vi "DistributedCSMModule.vi"(7 "Name(\"\" to use uuid)":string="Event CSM") -> ()   [LabVIEW 2020]
uses:
  <userlib>/_NEVSTOP/Communicable State Machine(CSM)/_Support/Common/Format Timestamp.vi
  <userlib>/_NEVSTOP/Communicable State Machine(CSM)/AdvanceAPI/CSM - Revert Arguments-Safe String.vi
  <userlib>/_NEVSTOP/Communicable State Machine(CSM)/_Support/Common/Trim Single line Text.vi
  <userlib>/_NEVSTOP/Communicable State Machine(CSM)/AdvanceAPI/CSM - Make String Arguments Safe.vi
  <userlib>/_NEVSTOP/Communicable State Machine(CSM)/AdvanceAPI/CSM - Break Down Multiple States String.vi
  <userlib>/_NEVSTOP/Communicable State Machine(CSM)/AdvanceAPI/CSM - Compact Multiple States.vi
  <userlib>/_NEVSTOP/Communicable State Machine(CSM)/AdvanceAPI/CSM - Keywords.vi
  <userlib>/_NEVSTOP/Communicable State Machine(CSM)/_Support/CSMQ/_CSMOFGV.vi
  <userlib>/_NEVSTOP/Communicable State Machine(CSM)/Communicable State Machine.lvlib
panel:
  out "State History":string
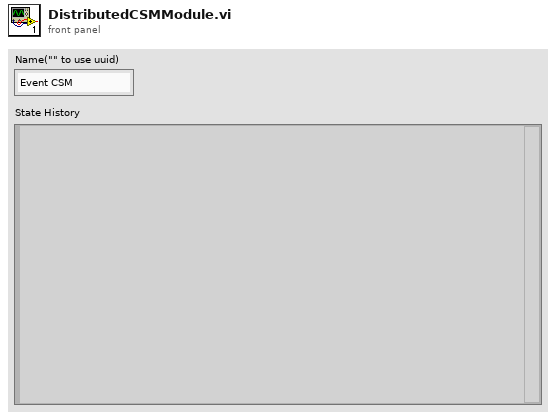
[diagram p1: front panel]
types:
  T1 = enum32{"Invalid", "Standard", "Closed", "Hidden", "Minimized", "Maximized"}
  T2 = enum32{"invalid app kind", "Development System", "Run Time System", "Student Edition", "Embedded LabVIEW", "Evaluation", "Custom"}
  T3 = typedef "Communicable State Machine.lvlib/_CSM_Response Source Message.ctl" = cluster{"‘State":string, "’Arguments":string, "’Error":errorcluster}
  T4 = cluster{"Current VI Reference":refnum<vi>, "Close Panel on Exit?":bool}
  T5 = cluster{"Core":cluster{"Current VI Reference":refnum<vi>, "Close Panel on Exit?":bool}, "Your Boolean data":bool, "Your string data":string}
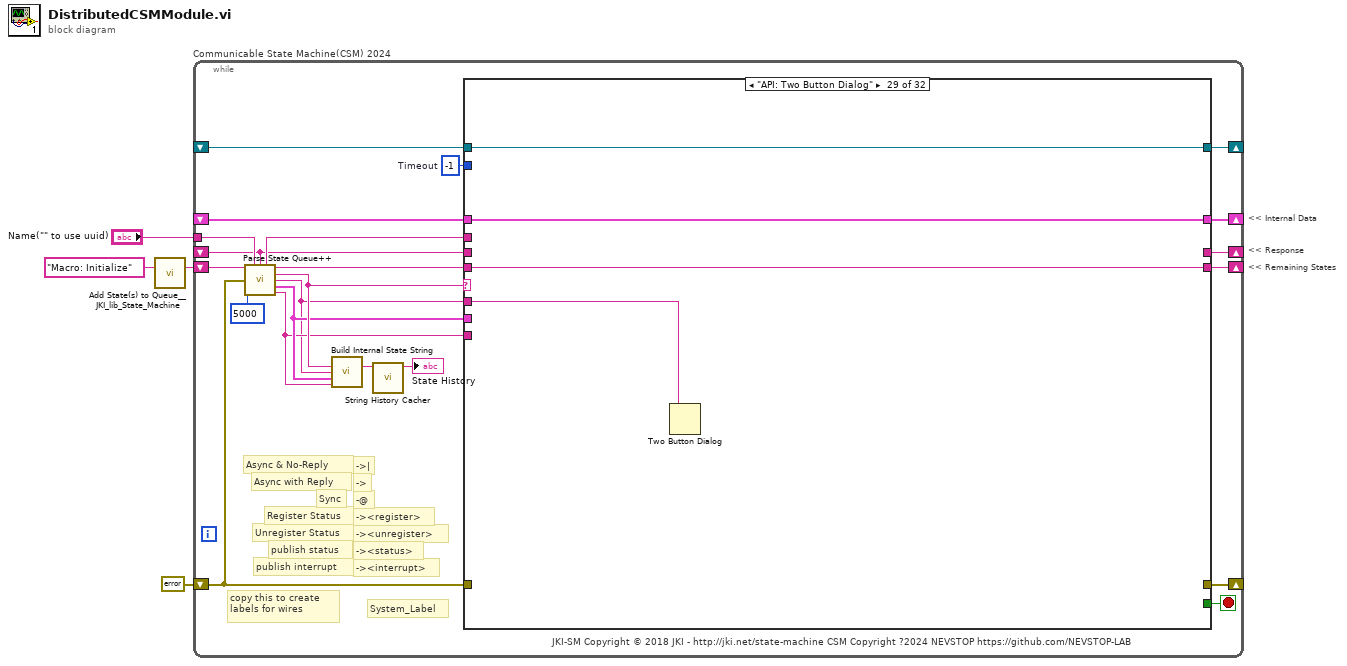
[diagram p0: block diagram]
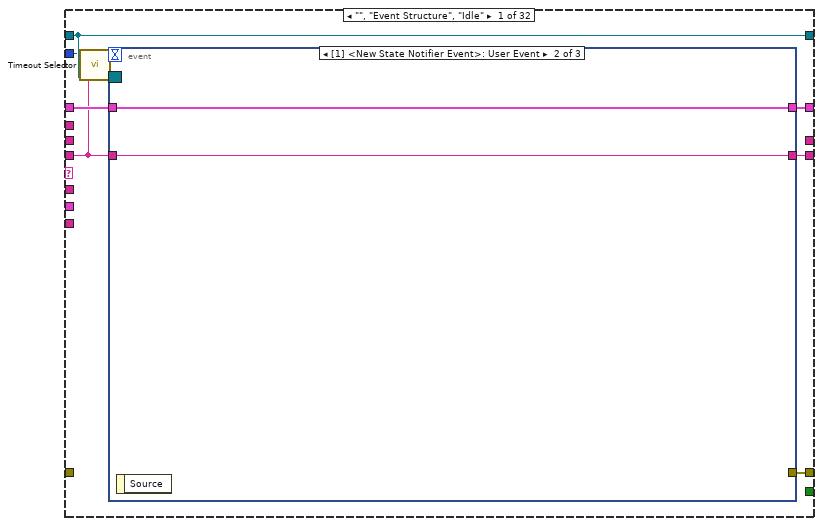
[diagram p2: hidden frame]
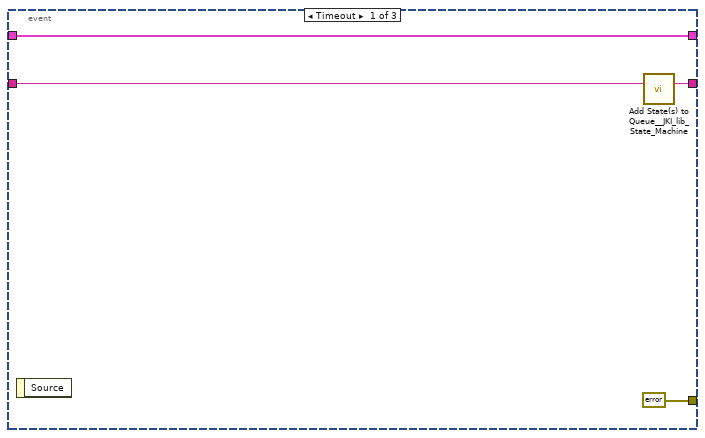
[diagram p3: hidden frame]
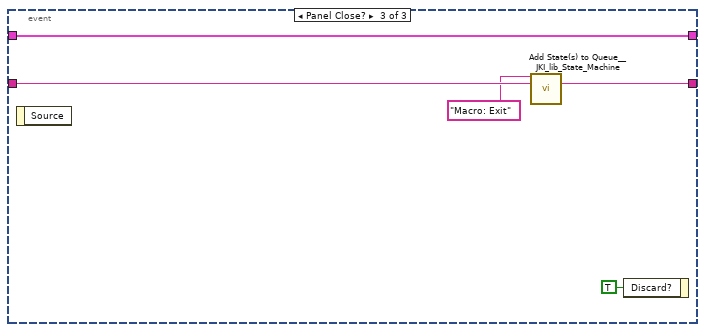
[diagram p4: hidden frame]
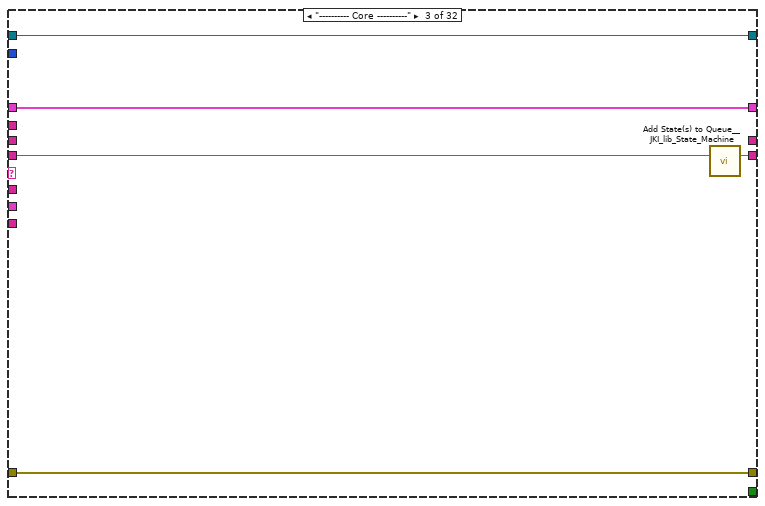
[diagram p6: hidden frame]
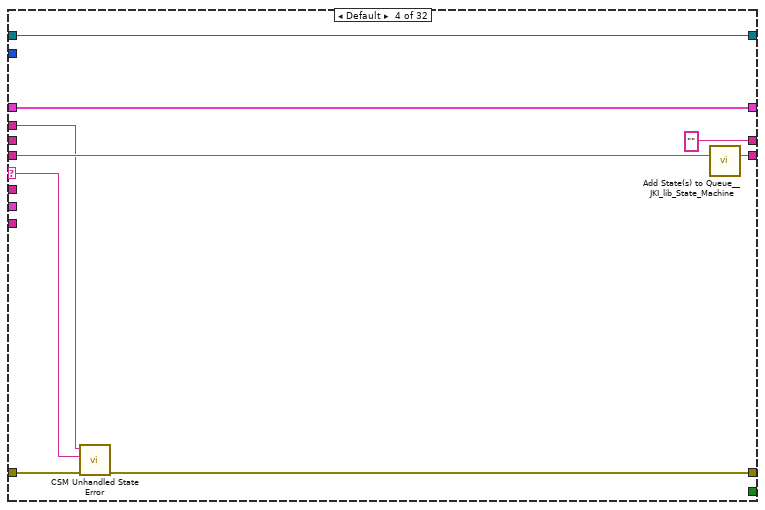
[diagram p7: hidden frame]
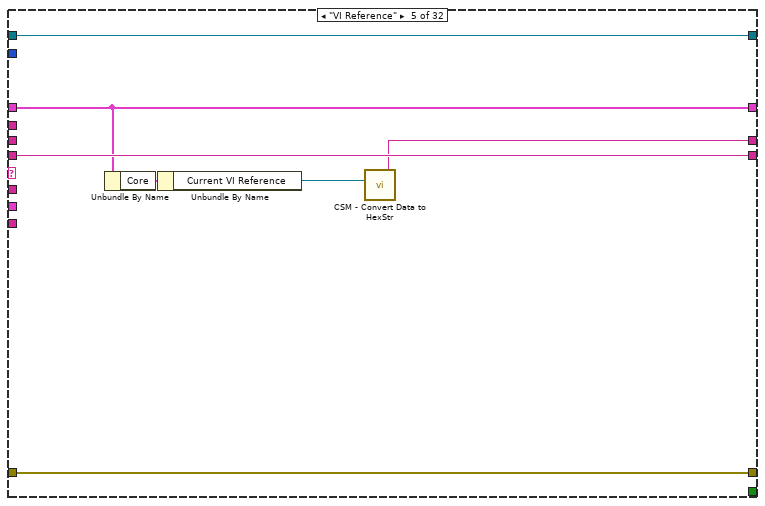
[diagram p8: hidden frame]
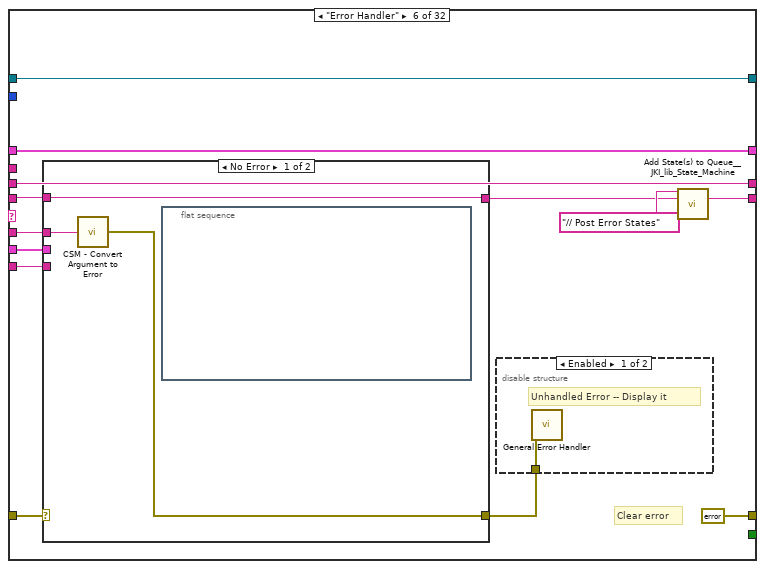
[diagram p9: hidden frame]
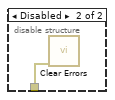
[diagram p10: hidden frame]
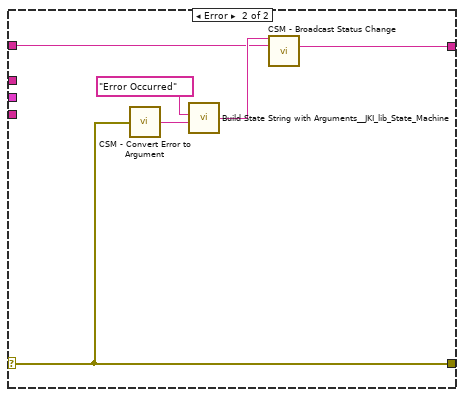
[diagram p11: hidden frame]
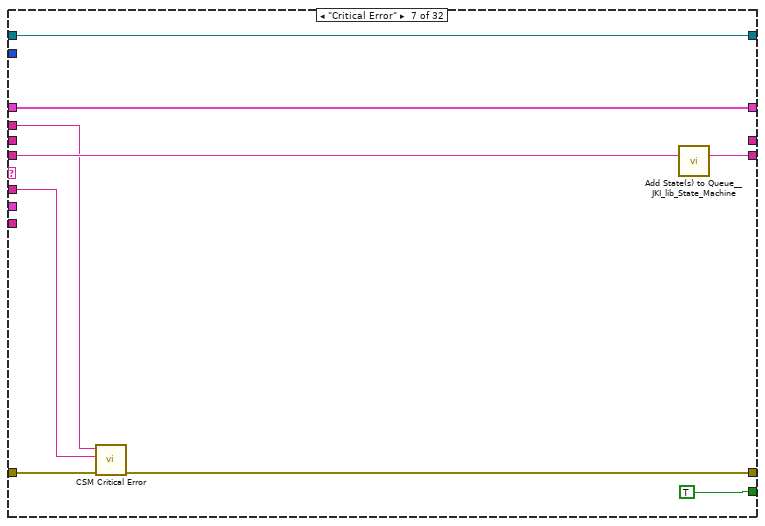
[diagram p12: hidden frame]
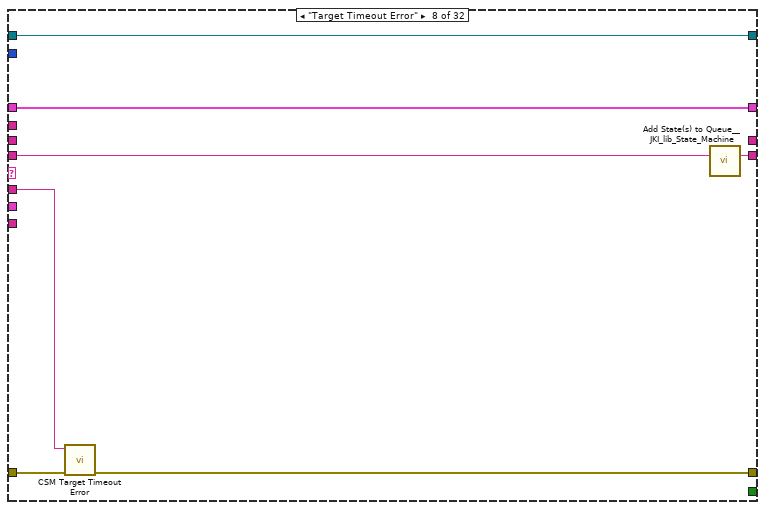
[diagram p13: hidden frame]
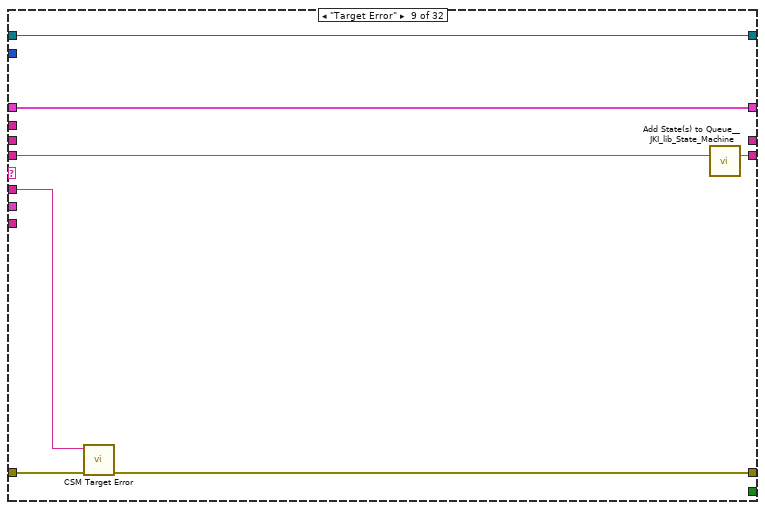
[diagram p14: hidden frame]
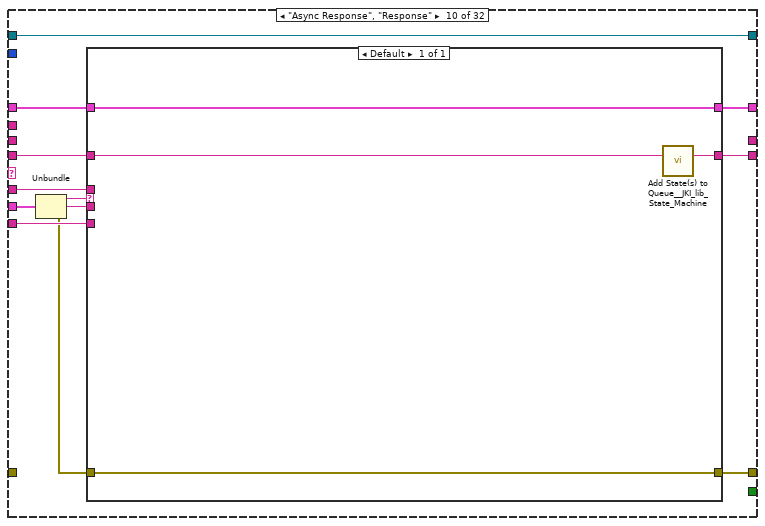
[diagram p15: hidden frame]
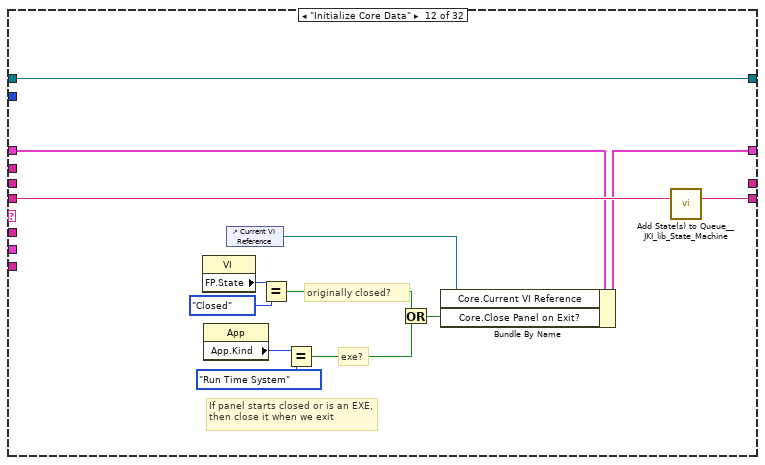
[diagram p17: hidden frame]
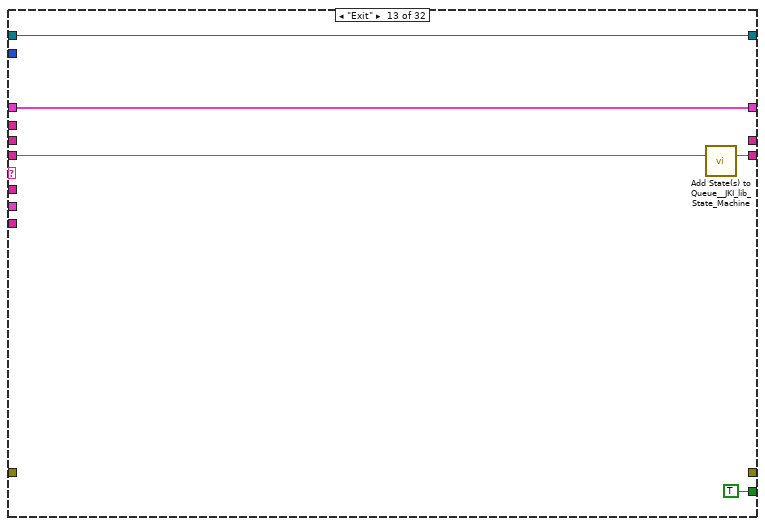
[diagram p18: hidden frame]
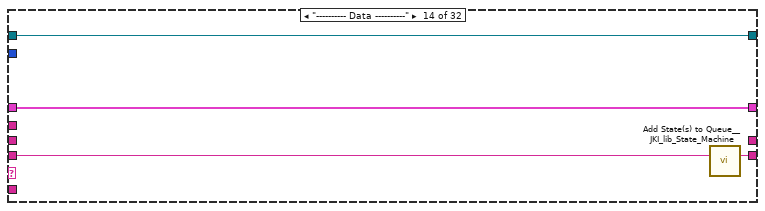
[diagram p19: hidden frame]
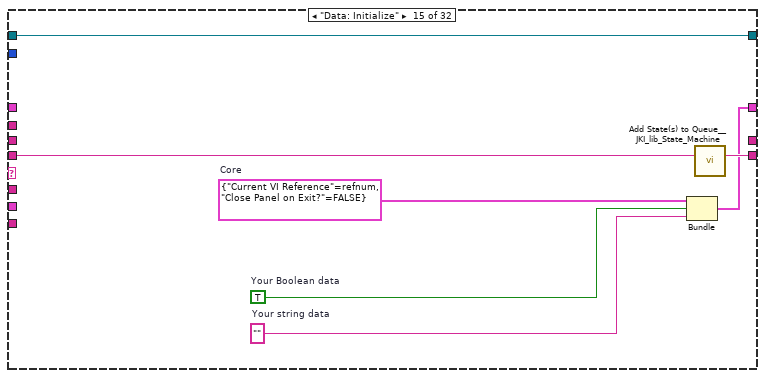
[diagram p20: hidden frame]
diagram:
  # "<< Internal Data"
  # "<< Response"
  # "<< Remaining States"
  n1 = call <vilib>:"Add State(s) to Queue__JKI_lib_State_Machine.vi"("State(s) in (\"\")"="Macro: Initialize" ("Init State(\"Macro: Initialize\")")) -> ("States Out"=w1:string)  [unwired: 14 in]
  n2 = while "Communicable State Machine(CSM) 2024" {
    shift-right: [w21] -> _
    shift-left: _ -> [w20]
    shift-right: [w24] -> _
    shift-left: errorcluster {"status"=FALSE, "code"=0, "source"=""} ("error out") -> [w18]
    shift-right: [w23] -> _
    shift-left: w1 -> [w25]
    tunnel: "Name(\"\" to use uuid)" -> [w13]
    shift-right: [w16] -> _
    shift-left: _ -> [w6]
    shift-right: [w15] -> _
    shift-left: _ -> [w14]
    stop <- w22 stop-if-true
    w19 = -1  # Timeout
    # "-><interrupt>"
    # "-><status>"
    # "-><unregister>"
    # "-><register>"
    # "-@"
    # "->"
    # "->|"
    # "publish interrupt"
    # "publish status"
    # "Unregister Status"
    # "Register Status"
    # "Sync"
    # "Async with Reply"
    # "Async & No-Reply"
    # "copy this to create labels for wires"
    # "System_Label"
    # "JKI-SM Copyright © 2018 JKI - http://jki.net/state-machine CSM Copyright ?2024 NEVSTOP https://github.com/NEVSTOP-LAB"
    n3 = call <userlib>:"Parse State Queue++.vi"("State Queue"=w25, "Name(\"\" to use uuid)"=w13, "Response Arguments"=w6, "Error In (no error)"=w18, "Response Timeout(5000ms)"=5000 ("Response Timeout(1000ms)")) -> ("Name Used"=w7:string, "Remaining States"=w26:string, "Current State"=w10:string, "Arguments"=w5:string, ">> Response Source Message >>"=w9:T3, ">> Source CSM >>"=w8:string)  [unwired: 5 in]
    n4 = call <userlib>:"Build Internal State String.vi"("State"=w10, "Arguments (\"\")"=w5, ">> Response Source Message >>"=w9, "Source (\"\")"=w8) -> ("State with Arguments"=w11:string)  [unwired: 11 in]
    n5 = call <userlib>:"String History Cacher.vi"("String"=w11) -> ("String Cache"=→"State History":string)  [unwired: 10 in]
    n6 = case shown="\"API: Two Button Dialog\"" w10 {
      selector: w10 -> [_ _ _ w56 _ _ _ _ _ _ _ _ _ _ _ _ _ _ _ _ _ _ _ _ _ _ _ _ _ _ _ _]
      tunnel: w26 -> [w27 w48 w53 w62 w68 w75 w101 w109 w116 w126 w135 w148 w153 w157 w164 w170 w174 w181 w185 w189 w193 w199 w211 w275 w280 w291 w294 w298 w302 w306 w310 w314]
      tunnel: w5 -> [_ _ _ _ _ w73 w97 w104 w112 w120 _ _ _ _ _ _ _ _ _ _ _ w195 w206 _ _ _ _ w295 w299 _ _ _]
      tunnel: w20 -> [w33 w47 w50 w60 w67 w81 w102 w107 w114 w124 w134 w142 w151 w155 _ w166 w172 w180 w184 w187 w191 w197 w208 w273 w278 w289 w293 w297 w301 w304 w308 w312]
      tunnel: [w32 _ w51 w54 w69 errorcluster {"status"=FALSE, "code"=0, "source"=""} ("error out") w94 w103 w110 w123 _ _ _ _ _ w167 _ w175 w183 _ _ w196 w209 _ _ _ _ _ _ _ _ _] -> w24
      tunnel: w18 -> [_ _ w51 w55 w69 w79 w95 w105 w111 _ _ _ _ _ _ _ _ _ _ _ _ _ _ _ _ _ _ _ _ _ _ _]
      tunnel: [w34 w48 w52 w61 w68 w77 w100 w108 w115 w127 w135 w147 w152 w156 w163 w169 w173 w181 w185 w188 w192 w198 w210 w274 w279 w290 w294 w298 w302 w305 w309 w313] -> w23
      tunnel: [_ _ _ _ _ _ TRUE _ _ _ _ _ TRUE _ _ _ _ _ _ _ _ _ _ _ _ _ _ _ _ _ _ _] -> w22
      tunnel: [w31 w47 w50 w60 w67 w81 w102 w107 w114 w125 w134 w146 w151 w155 w162 w166 w172 w180 w184 w187 w191 w197 w208 w273 w278 w289 w293 w297 w301 w304 w308 w312] -> w21
      tunnel: w19 -> [w29 _ _ _ _ _ _ _ _ _ _ _ _ _ _ _ _ _ _ _ _ _ _ _ _ _ _ _ _ _ _ _]
      tunnel: w8 -> [_ _ _ _ _ w72 _ _ _ w121 _ _ _ _ _ _ _ _ _ _ _ _ _ _ _ _ _ _ _ _ _ _]
      tunnel: w9 -> [_ _ _ _ _ w71 _ _ _ w122 _ _ _ _ _ _ _ _ _ _ _ _ _ _ _ _ _ _ _ _ _ _]
      tunnel: [_ _ _ "" w63 w70 _ _ _ _ _ _ _ _ _ _ _ _ _ _ _ _ _ _ _ _ _ _ _ _ _ _] -> w16
      tunnel: [w30 w46 w49 w58 w66 w80 w98 w106 w113 w128 w133 w136 w149 w154 w158 w165 w171 w179 w182 w186 w190 w194 w205 w272 w276 w282 w292 w296 w300 w303 w307 w311] -> w15
      tunnel: w14 -> [w30 w46 w49 w58 w66 w80 w98 w106 w113 w128 w133 w136 w149 w154 w158 w165 w171 _ w182 w186 w190 w194 w205 w272 w276 w282 w292 w296 w300 w303 w307 w311]
      tunnel: w7 -> [_ _ _ w57 _ _ w96 _ _ _ _ _ _ _ _ _ _ w178 _ _ _ _ _ _ _ _ _ _ _ _ _ _]
      tunnel: w6 -> [_ _ _ _ _ w70 _ _ _ _ _ _ _ _ _ _ _ _ _ _ _ _ _ _ _ _ _ _ _ _ _ _]
      frame "", "Event Structure", "Idle" {
        n7 = call <userlib>:"Timeout Selector.vi"("Remaining States"=w27, "Timeout Expected"=w29) -> ("Timeout"=w28:i32)  [unwired: 5 in]
        n8 = event shown="[1] <New State Notifier Event>: User Event" {
          selector: w30 -> [_ _ _]
          dyn-events: _ -> [_ _ _]
          timeout: w28 -> [_ _ _]
          tunnel: w27 -> [w38 w39 w45]
          tunnel: [w37 w39 w44] -> w34
          tunnel: w33 -> [w36 w40 w43]
          tunnel: [errorcluster {"status"=FALSE, "code"=0, "source"=""} ("error out") _ _] -> w32
          tunnel: [w36 w40 w43] -> w31
          event Timeout {
            n9 = event-data() -> ()  [unwired: 1 in, 1 out]
            n10 = call <vilib>:"Add State(s) to Queue__JKI_lib_State_Machine.vi"("State(s) in (\"\")"=w38) -> ("States Out"=w37:string)  [unwired: 14 in]
          }
          event User Event {
            n11 = event-data() -> ()  [unwired: 1 in, 1 out]
          }
          event Panel Close? {
            n12 = event-data() -> ()  [unwired: 1 in, 1 out]
            n13 = call <vilib>:"Add State(s) to Queue__JKI_lib_State_Machine.vi"("State(s) in Front (\"\")"="Macro: Exit", "State(s) in (\"\")"=w45) -> ("States Out"=w44:string)  [unwired: 13 in]
            n14 = event-data("Discard?"=TRUE) -> ()  [unwired: 1 in, 1 out]
          }
        }
      }
      frame "CSM Documentation" {
      }
      frame "---------- Core ----------" {
        n15 = call <vilib>:"Add State(s) to Queue__JKI_lib_State_Machine.vi"("State(s) in (\"\")"=w53) -> ("States Out"=w52:string)  [unwired: 14 in]
      }
      frame Default {
        n16 = call <userlib>:"CSM Unhandled State Error.vi"("error in (no error)"=w55, "Current State"=w56, "CSM Name"=w57) -> ("error out"=w54:errorcluster)  [unwired: 8 in]
        n17 = call <vilib>:"Add State(s) to Queue__JKI_lib_State_Machine.vi"("State(s) in (\"\")"=w62) -> ("States Out"=w61:string)  [unwired: 14 in]
      }
      frame "VI Reference" {
        n18 = Unbundle By Name(w67) -> ("Core"=w65:T4)
        n19 = Unbundle By Name(w65) -> ("Current VI Reference"=w64:refnum<vi>)
        n20 = call <userlib>:"CSM - Convert Data to HexStr.vi"("Variant"=w64) -> ("HEX String (0-9,A-F)"=w63:string)  [unwired: 8 in]
      }
      frame "Error Handler" {
        # "Clear error"
        n21 = case shown="No Error" w79 {
          selector: w79 -> [_ w88]
          tunnel: [w86 w90] -> w76
          tunnel: w75 -> [w86 w89]
          tunnel: [w85 w88] -> w74
          tunnel: w73 -> [w87 _]
          tunnel: w72 -> [_ _]
          tunnel: w71 -> [_ _]
          frame No Error {
            n22 = call <userlib>:"CSM - Convert Argument to Error.vi"("Argument"=w87) -> ("error"=w85:errorcluster)  [unwired: 4 in]
            n23 = flat-sequence {
              frame #0 {
              }
            }
          }
          frame Error {
            n24 = call <userlib>:"CSM - Convert Error to Argument.vi"("error in (no error)"=w88) -> ("Arguments"=w92:string)  [unwired: 4 in]
            n25 = call <vilib>:"Build State String with Arguments__JKI_lib_State_Machine.vi"("Arguments (\"\")"=w92, "State"="Error Occurred" ("Status with Arguments")) -> ("State with Arguments"=w91:string)  [unwired: 4 in]
            n26 = call <userlib>:"CSM - Broadcast Status Change.vi"("Status with Arguments"=w91, "State Queue"=w89) -> ("Remaining States"=w90:string)  [unwired: 13 in]
          }
        }
        n27 = disable-structure shown="Enabled" {
          disable-tunnel: w74 -> [w83 w84]
          frame Enabled {
            # "Unhandled Error -- Display it"
            n28 = call <vilib>:"General Error Handler.vi"("error in (no error)"=w83) -> ()  [unwired: 10 in, 5 out]
          }
          frame Disabled {
            n29 = call <vilib>:"Clear Errors.vi"("error in (no error)"=w84) -> ()  [unwired: 5 in, 2 out]
          }
        }
        n30 = call <vilib>:"Add State(s) to Queue__JKI_lib_State_Machine.vi"("State(s) in Front (\"\")"="// Post Error States", "State(s) in (\"\")"=w76) -> ("States Out"=w77:string)  [unwired: 13 in]
      }
      frame "Critical Error" {
        n31 = call <userlib>:"CSM Critical Error.vi"("error in (no error)"=w95, "Arugments(as Reason)"=w97, "CSM Name"=w96) -> ("error out"=w94:errorcluster)  [unwired: 8 in]
        n32 = call <vilib>:"Add State(s) to Queue__JKI_lib_State_Machine.vi"("State(s) in (\"\")"=w101) -> ("States Out"=w100:string)  [unwired: 14 in]
      }
      frame "Target Timeout Error" {
        n33 = call <userlib>:"CSM Target Timeout Error.vi"("error in (no error)"=w105, "Arguments(as CSM Name)"=w104) -> ("error out"=w103:errorcluster)  [unwired: 9 in]
        n34 = call <vilib>:"Add State(s) to Queue__JKI_lib_State_Machine.vi"("State(s) in (\"\")"=w109) -> ("States Out"=w108:string)  [unwired: 14 in]
      }
      frame "Target Error" {
        n35 = call <userlib>:"CSM Target Error.vi"("error in (no error)"=w111, "Arguments(as CSM Name)"=w112) -> ("error out"=w110:errorcluster)  [unwired: 9 in]
        n36 = call <vilib>:"Add State(s) to Queue__JKI_lib_State_Machine.vi"("State(s) in (\"\")"=w116) -> ("States Out"=w115:string)  [unwired: 14 in]
      }
      frame "Async Response", "Response" {
        n37 = Unbundle(w122) -> ("‘State"=w119:string, "’Arguments"=w118:string, "’Error"=w117:errorcluster)
        n38 = case shown="Default" w119 {
          tunnel: [w129] -> w127
          tunnel: w126 -> [w130]
          tunnel: [w132] -> w125
          tunnel: w124 -> [w132]
          tunnel: [w131] -> w123
          tunnel: w117 -> [w131]
          tunnel: w121 -> [_]
          tunnel: w120 -> [_]
          tunnel: w118 -> [_]
          frame Default {
            n39 = call <vilib>:"Add State(s) to Queue__JKI_lib_State_Machine.vi"("State(s) in (\"\")"=w130) -> ("States Out"=w129:string)  [unwired: 14 in]
          }
        }
      }
      frame "Async Message Posted" {
      }
      frame "Initialize Core Data" {
        # "originally closed?"
        # "exe?"
        # "If panel starts closed or is an EXE, then close it when we exit"
        n40 = property class="VI"() -> ("FP.State"=w139:T1)  [unwired: 2 in, 2 out]
        n41 = property class="App"() -> ("App.Kind"=w145:T2)  [unwired: 2 in, 2 out]
        n42 = control-ref of="Current VI Reference"() -> (w140:refnum<vi>)
        n43 = Equal?(x=w139, y=T1."Closed" ("Front Panel Window:State")) -> (x = y?=w137:bool)
        n44 = Equal?(x=w145, y=T2."Run Time System" ("Application:Kind")) -> (x = y?=w143:bool)
        n45 = Or(x=w137, y=w143) -> (x .or. y?=w141:bool)
        n46 = Bundle By Name(cluster=w142, "Core.Current VI Reference"=w140, "Core.Close Panel on Exit?"=w141) -> (w146:T5)
        n47 = call <vilib>:"Add State(s) to Queue__JKI_lib_State_Machine.vi"("State(s) in (\"\")"=w148) -> ("States Out"=w147:string)  [unwired: 14 in]
      }
      frame "Exit" {
        n48 = call <vilib>:"Add State(s) to Queue__JKI_lib_State_Machine.vi"("State(s) in (\"\")"=w153) -> ("States Out"=w152:string)  [unwired: 14 in]
      }
      frame "---------- Data ----------" {
        n49 = call <vilib>:"Add State(s) to Queue__JKI_lib_State_Machine.vi"("State(s) in (\"\")"=w157) -> ("States Out"=w156:string)  [unwired: 14 in]
      }
      frame "Data: Initialize" {
        w159 = T4 {"Current VI Reference"=refnum, "Close Panel on Exit?"=FALSE}  # Core
        w161 = TRUE  # Your Boolean data
        w160 = ""  # Your string data
        n50 = Bundle("Core"=w159, "Your Boolean data"=w161, "Your string data"=w160) -> (w162:T5)  [unwired: 1 in]
        n51 = call <vilib>:"Add State(s) to Queue__JKI_lib_State_Machine.vi"("State(s) in (\"\")"=w164) -> ("States Out"=w163:string)  [unwired: 14 in]
      }
      frame "Data: Cleanup" {
        n52 = Unbundle By Name(w166) -> ("Core.Current VI Reference"=w168:refnum<vi>)
        n53 = Close Reference(reference=w168) -> (error out=w167:errorcluster)  [unwired: 1 in]
        n54 = call <vilib>:"Add State(s) to Queue__JKI_lib_State_Machine.vi"("State(s) in (\"\")"=w170) -> ("States Out"=w169:string)  [unwired: 14 in]
      }
      frame "---------- Events ----------" {
        n55 = call <vilib>:"Add State(s) to Queue__JKI_lib_State_Machine.vi"("State(s) in (\"\")"=w174) -> ("States Out"=w173:string)  [unwired: 14 in]
      }
      frame "Events: Register" {
        n56 = call <userlib>:"CSM - Get New State Notifier Event.vi"("Name(\"\" to use uuid) in"=w178) -> ("Error out"=w176:errorcluster, "New State Notifier Event"=w177:refnum<user-event>)  [unwired: 9 in]
        n57 = register-events(error in=w176, w177) -> (reference out=w179:refnum<event-registration>, error out=w175:errorcluster)  [unwired: 1 in]
      }
      frame "Events: Unregister" {
        n58 = Unregister For Events(event registration refnum=w182) -> (error out=w183:errorcluster)  [unwired: 1 in]
      }
      frame "---------- UI ----------" {
        n59 = call <vilib>:"Add State(s) to Queue__JKI_lib_State_Machine.vi"("State(s) in (\"\")"=w189) -> ("States Out"=w188:string)  [unwired: 14 in]
      }
      frame "UI: Initialize" {
        n60 = call <vilib>:"Add State(s) to Queue__JKI_lib_State_Machine.vi"("State(s) in (\"\")"=w193) -> ("States Out"=w192:string)  [unwired: 14 in]
      }
      frame "UI: Cursor Set" {
        # "Argument"
        n61 = disable-structure shown="Default" {
          disable-tunnel: [w201 w204] -> w196
          disable-tunnel: w195 -> [w200 _]
          frame condition #0 (active) {
            n62 = case shown="\"Idle\", Default" w200 {
              tunnel: [w202 w203] -> w201
              frame "Idle", Default {
                n63 = call <vilib>:"Unset Busy.vi"() -> ("error out"=w202:errorcluster)  [unwired: 11 in]
              }
              frame "Busy" {
                n64 = call <vilib>:"Set Busy.vi"() -> ("error out"=w203:errorcluster)  [unwired: 10 in, 1 out]
              }
            }
          }
          frame condition #1 {
          }
        }
        n65 = call <vilib>:"Add State(s) to Queue__JKI_lib_State_Machine.vi"("State(s) in (\"\")"=w199) -> ("States Out"=w198:string)  [unwired: 14 in]
      }
      frame "UI: Front Panel State" {
        # "Argument"
        n66 = Unbundle By Name(w208) -> ("Core.Current VI Reference"=w207:refnum<vi>)
        n67 = case shown="\"Minimize\", \"Minimized\"" w206 {
          tunnel: [w218 w231 w242 w254 w266] -> w209
          tunnel: w207 -> [w217 w229 w241 w253 w265]
          frame "Open", "Standard", Default {
            w212 = T1."Standard" ("State")
            n68 = property class="VI"(reference=w217) -> (reference out=w215:refnum<vi>, error out=w216:errorcluster, "FP.State"=w214:T1)  [unwired: 1 in]
            n69 = Not Equal?(x=w214, y=w212) -> (x != y?=w213:bool)
            n70 = case shown="True" w213 {
              tunnel: [w222 w224] -> w218
              tunnel: w216 -> [w221 w224]
              tunnel: w215 -> [w220 _]
              tunnel: w212 -> [w219 _]
              frame True {
                n71 = invoke class="VI" method="FP.Open"(reference=w220, error in=w221, "Activate"=TRUE, "State"=w219) -> (error out=w222:errorcluster)  [unwired: 1 in, 4 out]
              }
              frame False {
              }
            }
          }
          frame "Close", "Closed" {
            n72 = property class="VI"(reference=w229) -> (reference out=w228:refnum<vi>, error out=w230:errorcluster, "FP.State"=w226:T1)  [unwired: 1 in]
            n73 = Not Equal?(x=w226, y=T1."Closed" ("Front Panel Window:State")) -> (x != y?=w225:bool)
            n74 = case shown="True" w225 {
              tunnel: [w232 w235] -> w231
              tunnel: w230 -> [w232 w234]
              tunnel: w228 -> [_ w233]
              frame False {
              }
              frame True {
                n75 = invoke class="VI" method="FP.Close"(reference=w233, error in=w234) -> (error out=w235:errorcluster)  [unwired: 1 in, 2 out]
              }
            }
          }
          frame "Hidden", "Hide" {
            w236 = T1."Hidden" ("State")
            n76 = property class="VI"(reference=w241) -> (reference out=w239:refnum<vi>, error out=w240:errorcluster, "FP.State"=w238:T1)  [unwired: 1 in]
            n77 = Not Equal?(x=w238, y=w236) -> (x != y?=w237:bool)
            n78 = case shown="True" w237 {
              tunnel: [w246 w247] -> w242
              tunnel: w240 -> [w245 w247]
              tunnel: w239 -> [w244 _]
              tunnel: w236 -> [w243 _]
              frame True {
                n79 = invoke class="VI" method="FP.Open"(reference=w244, error in=w245, "State"=w243) -> (error out=w246:errorcluster)  [unwired: 2 in, 4 out]
              }
              frame False {
              }
            }
          }
          frame "Minimize", "Minimized" {
            w248 = T1."Minimized" ("State")
            n80 = property class="VI"(reference=w253) -> (reference out=w251:refnum<vi>, error out=w252:errorcluster, "FP.State"=w250:T1)  [unwired: 1 in]
            n81 = Not Equal?(x=w250, y=w248) -> (x != y?=w249:bool)
            n82 = case shown="False" w249 {
              tunnel: [w258 w259] -> w254
              tunnel: w252 -> [w257 w259]
              tunnel: w251 -> [w256 _]
              tunnel: w248 -> [w255 _]
              frame True {
                n83 = invoke class="VI" method="FP.Open"(reference=w256, error in=w257, "State"=w255) -> (error out=w258:errorcluster)  [unwired: 2 in, 4 out]
              }
              frame False {
              }
            }
          }
          frame "Maximize", "Maximized" {
            w260 = T1."Maximized" ("State")
            n84 = property class="VI"(reference=w265) -> (reference out=w263:refnum<vi>, error out=w264:errorcluster, "FP.State"=w262:T1)  [unwired: 1 in]
            n85 = Not Equal?(x=w262, y=w260) -> (x != y?=w261:bool)
            n86 = case shown="True" w261 {
              tunnel: [w270 w271] -> w266
              tunnel: w264 -> [w269 w271]
              tunnel: w263 -> [w268 _]
              tunnel: w260 -> [w267 _]
              frame True {
                n87 = invoke class="VI" method="FP.Open"(reference=w268, error in=w269, "State"=w267) -> (error out=w270:errorcluster)  [unwired: 2 in, 4 out]
              }
              frame False {
              }
            }
          }
        }
        n88 = call <vilib>:"Add State(s) to Queue__JKI_lib_State_Machine.vi"("State(s) in (\"\")"=w211) -> ("States Out"=w210:string)  [unwired: 14 in]
      }
      frame "---------- Macro ----------" {
        n89 = call <vilib>:"Add State(s) to Queue__JKI_lib_State_Machine.vi"("State(s) in (\"\")"=w275) -> ("States Out"=w274:string)  [unwired: 14 in]
      }
      frame "Macro: Initialize" {
        w277 = "Data: Initialize\nInitialize Core Data\nEvents: Register\nUI: Initialize\nUI: Front Panel State >> Open"  # Data: Initialize Initialize Core Data Events: Register UI: Initialize UI: Front Panel State >> Open
        n90 = call <vilib>:"Add State(s) to Queue__JKI_lib_State_Machine.vi"("State(s) in Front (\"\")"=w277, "State(s) in (\"\")"=w280) -> ("States Out"=w279:string)  [unwired: 13 in]
      }
      frame "Macro: Exit" {
        n91 = Unbundle By Name(w289) -> ("Core.Close Panel on Exit?"=w288:bool)
        n92 = Select(t="UI: Front Panel State >> Close", s=w288, f="") -> (s? t:f=w285:string)
        n93 = call <vilib>:"Add State(s) to Queue__JKI_lib_State_Machine.vi"("State(s) in Front (\"\")"="//Exit Sub-Modules ", "State(s) in (\"\")"=w285, "State(s) at Back (\"\")"="Data: Cleanup\nEvents: Unregister\nExit") -> ("States Out"=w283:string)  [unwired: 12 in]
        n94 = call <vilib>:"Add State(s) to Queue__JKI_lib_State_Machine.vi"("State(s) in Front (\"\")"=w283, "State(s) in (\"\")"=w291) -> ("States Out"=w290:string)  [unwired: 13 in]
      }
      frame "---------- API ----------" {
      }
      frame "API: One Button Dialog" {
        n95 = One Button Dialog(message=w295) -> ()  [unwired: 1 in, 1 out]
      }
      frame "API: Two Button Dialog" {
        n96 = Two Button Dialog(message=w299) -> ()  [unwired: 2 in, 1 out]
      }
      frame "---------- Action ----------" {
        n97 = call <vilib>:"Add State(s) to Queue__JKI_lib_State_Machine.vi"("State(s) in (\"\")"=w306) -> ("States Out"=w305:string)  [unwired: 14 in]
      }
      frame "Action: action1" {
        n98 = call <vilib>:"Add State(s) to Queue__JKI_lib_State_Machine.vi"("State(s) in (\"\")"=w310) -> ("States Out"=w309:string)  [unwired: 14 in]
      }
      frame "Action: action2" {
        n99 = call <vilib>:"Add State(s) to Queue__JKI_lib_State_Machine.vi"("State(s) in (\"\")"=w314) -> ("States Out"=w313:string)  [unwired: 14 in]
      }
    }
  }
